vi "Abort Copy Blob.vi"(7 "Copy ID":string, 8 "error in (no error)":errorcluster, 9 "Blob":string, 10 "Container":string, 11 "Azure Session in":refnum<class "Session.lvclass">) -> (0 "error out":errorcluster, 3 "Azure Session out":refnum<class "Session.lvclass">)   [LabVIEW 2015, in "NI_Azure_Blob.lvlib"]
doc: "Aborts a pending Copy Blob operation, and leaves a destination blob with zero length and full metadata."
uses:
  NI_Azure_Blob.lvlib
  Core/Session/Session.lvclass
  Core/Name Value Pair.ctl
  Core/Session/Session.lvclass/Session.ctl
  Core/Session/Write Request Parameters.vi
  Core/Session/Write URL Suffix.vi
  Core/Session/Write HTTP Verb.vi
  Core/Session/Write Request Headers.vi
  Core/NI_Azure_Core.lvlib
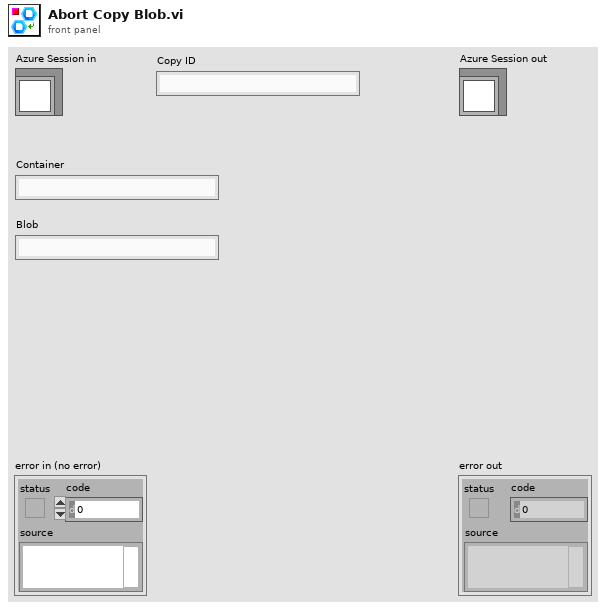
[diagram p1: front panel]
types:
  T1 = typedef "NI_Azure_Core.lvlib/Name Value Pair.ctl" = cluster{"name":string, "value":string}
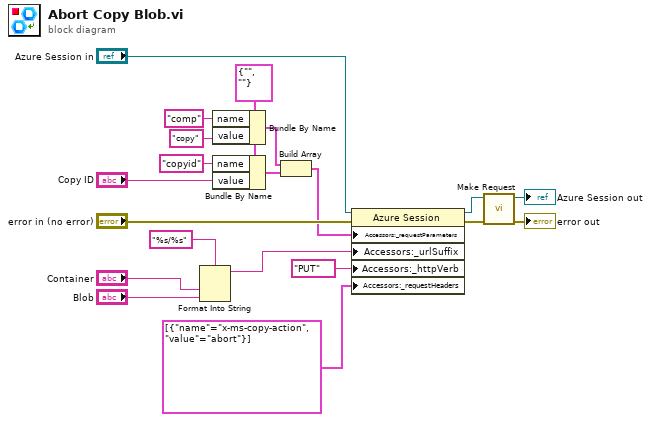
[diagram p0: block diagram]
diagram:
  w7 = T1 {"name"="", "value"=""} ("Name Value Pair")
  n1 = Format Into String(format string="%s/%s", "Container", "Blob") -> (resulting string=w11:string)  [unwired: 2 in, 1 out]
  n2 = Bundle By Name(cluster=w7, "name"="comp", "value"="copy") -> (w16:T1)
  n3 = Bundle By Name(cluster=w7, "name"="copyid", "value"="Copy ID") -> (w6:T1)
  n4 = Build Array(w16, w6) -> (w12:T1[])
  n5 = property class="Azure Session"(reference="Azure Session in", error in="error in (no error)", "Accessors:_requestParameters"=w12, "Accessors:_urlSuffix"=w11, "Accessors:_httpVerb"="PUT" ("HTTP-Verb"), "Accessors:_requestHeaders"=T1[] [{"name"="x-ms-copy-action", "value"="abort"}] ("_requestHeaders")) -> (reference out=w13:refnum<class "Session.lvclass">, error out=w14:errorcluster)
  n6 = call "Make Request.vi"("error in (no error)"=w14, "Session in"=w13) -> ("error out"=→"error out":errorcluster, "Session out"=→"Azure Session out":refnum<class "Session.lvclass">)  [unwired: 7 in, 1 out]
